vi "DeCoF example.vi"() -> ()   [LabVIEW 2013]
panel:
  out "uses DHCP":bool
  out "ip-address":string
  out "uptime (s)":i32
  out "system-label":string
  out "serial number":string
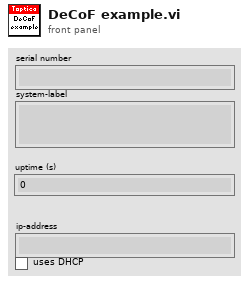
[diagram p1: front panel]
types:
  T1 = enum16{"Left Button", "Center Button", "Right Button", "Window Close"}
  T2 = typedef "DeCoF connection.ctl" = cluster{"TCP/IP":bool, "VISA":refnum<visa-resource-name>, "TCP/IP ID":refnum<k5>}
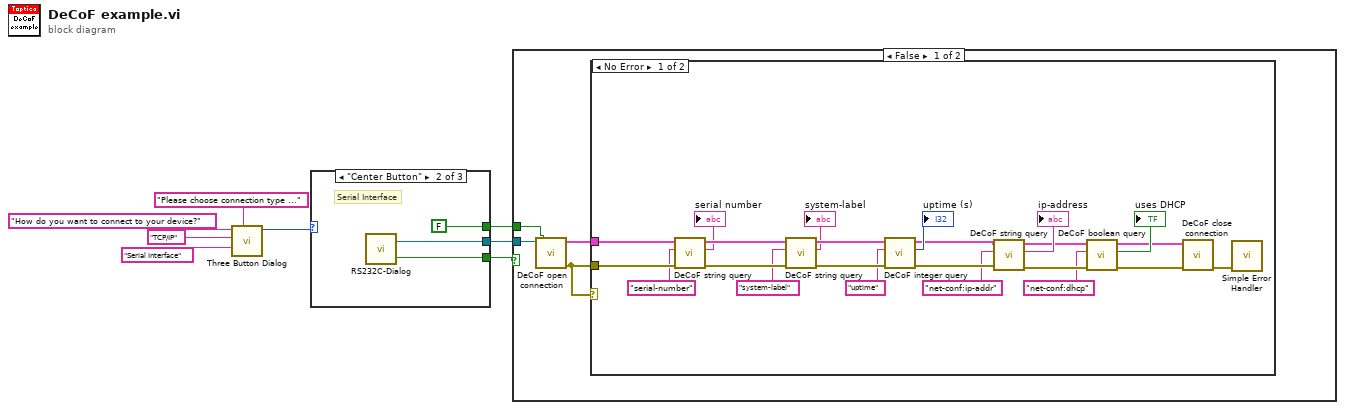
[diagram p0: block diagram]
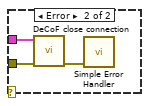
[diagram p2: hidden frame]
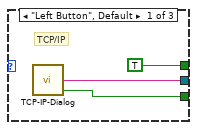
[diagram p4: hidden frame]
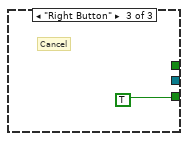
[diagram p5: hidden frame]
diagram:
  n1 = call <vilib>:"Three Button Dialog.vi"("Window Title (\"\")"="Please choose connection type ..." ("Window Title (\"\")"), "Center Button Text (\"No\")"="Serial Interface" ("Center Button Text (\"No\")"), "Left Button Text (\"Yes\")"="TCP/IP" ("Left Button Text (\"Yes\")"), "message"="How do you want to connect to your device?") -> ("Which Button?"=w4:T1)  [unwired: 7 in]
  n2 = case shown="\"Center Button\"" w4 {
    tunnel: [w11 w14 _] -> w3
    tunnel: [TRUE FALSE _] -> w2
    tunnel: [w9 w12 TRUE] -> w1
    frame "Left Button", Default {
      # "TCP/IP"
      n3 = call "TCP-IP-Dialog.vi"() -> ("IP address+ port"=w11:string, "cancelled"=w9:bool)  [unwired: 2 in, 1 out]
    }
    frame "Center Button" {
      # "Serial Interface"
      n4 = call "RS232C-Dialog.vi"() -> ("cancelled"=w12:bool, "VISA resource name"=w14:refnum<visa-resource-name>)
    }
    frame "Right Button" {
      # "Cancel"
    }
  }
  n5 = case shown="False" w1 {
    tunnel: w3 -> [w17 _]
    tunnel: w2 -> [w16 _]
    frame False {
      n6 = call "DeCoF open connection.vi"("TCP?"=w16, "address"=w17) -> ("error out"=w18:errorcluster, "Conncection ID out"=w19:T2)  [unwired: 4 in]
      n7 = case shown="No Error" w18 {
        tunnel: w18 -> [w42 w44]
        tunnel: w19 -> [w41 w45]
        frame No Error {
          n8 = call "DeCoF string query.vi"("error in"=w42, "param-name"="serial-number", "Conncection ID in"=w41) -> ("error out"=w39:errorcluster, "value"=→"serial number":string, "Conncection ID out"=w40:T2)  [unwired: 2 in]
          n9 = call "DeCoF string query.vi"("error in"=w39, "param-name"="system-label", "Conncection ID in"=w40) -> ("error out"=w37:errorcluster, "value"=→"system-label":string, "Conncection ID out"=w38:T2)  [unwired: 2 in]
          n10 = call "DeCoF integer query.vi"("error in"=w37, "param-name"="uptime", "Conncection ID in"=w38) -> ("error out"=w29:errorcluster, "value"=→"uptime (s)":i32, "Conncection ID out"=w30:T2)  [unwired: 2 in]
          n11 = call "DeCoF string query.vi"("error in"=w29, "param-name"="net-conf:ip-addr", "Conncection ID in"=w30) -> ("error out"=w25:errorcluster, "value"=→"ip-address":string, "Conncection ID out"=w26:T2)  [unwired: 2 in]
          n12 = call "DeCoF boolean query.vi"("error in"=w25, "param-name"="net-conf:dhcp", "Conncection ID in"=w26) -> ("error out"=w21:errorcluster, "value"=→"uses DHCP":bool, "Conncection ID out"=w22:T2)  [unwired: 2 in]
          n13 = call "DeCoF close connection.vi"("error in (no error)"=w21, "Connection ID in"=w22) -> ("error out"=w20:errorcluster)  [unwired: 4 in, 1 out]
          n14 = call <vilib>:"Simple Error Handler.vi"("error in (no error)"=w20) -> ()  [unwired: 4 in, 5 out]
        }
        frame Error {
          n15 = call "DeCoF close connection.vi"("error in (no error)"=w44, "Connection ID in"=w45) -> ("error out"=w43:errorcluster)  [unwired: 4 in, 1 out]
          n16 = call <vilib>:"Simple Error Handler.vi"("error in (no error)"=w43) -> ()  [unwired: 4 in, 5 out]
        }
      }
    }
    frame True {
      # "cancelled"
    }
  }
